vi "MultiTaskLassoCV.vi"(8 "error in":errorcluster) -> (0 "error out":errorcluster, 3 "out":refnum<class "MultiTaskLassoCV.lvclass">)   [LabVIEW 2020]
doc: "Multi-task Lasso model trained with L1/L2 mixed-norm as regularizer.\n\n See glossary entry for :term:`cross-validation estimator`.\n\n The optimization objective for MultiTaskLasso is::\n\n (1 / (2 * n_samples)) * ||Y - XW||^Fro_2 + alpha * ||W||_21\n\n Where::\n\n ||W||_21 = \\sum_i \\sqrt{\\sum_j w_{ij}^2}\n\n i.e. the sum of norm of each row.\n\n Read more in the :ref:`User Guide <multi_task_lasso>`.\n\n .. versionadded:: 0.15\n\n Parameters\n ----------\n eps : float, default=1e-3\n Length of the path. ``eps=1e-3`` means that\n ``alpha_min / alpha_max = 1e-3``.\n\n n_alphas : int, default=100\n Number of alphas along the regularization path.\n\n alphas : array-like, default=None\n List of alphas where to compute the models.\n If not provided, set automatically.\n\n fit_intercept : bool, default=True\n Whether to calculate the intercept for this model. If set\n to false, no intercept will be used in calculations\n (i.e. data is expected to be centered).\n\n normalize : bool, default=False\n This parameter is ignored when ``fit_intercept`` is set to False.\n If True, the regressors X will be normalized before regression by\n subtracting the mean and dividing by the l2-norm.\n If you wish to standardize, please use\n :class:`~sklearn.preprocessing.StandardScaler` before calling ``fit``\n on an estimator with ``normalize=False``.\n\n max_iter : int, default=1000\n The maximum number of iterations.\n\n tol : float, default=1e-4\n The tolerance for the optimization: if the updates are\n smaller than ``tol``, the optimization code checks the\n dual gap for optimality and continues until it is smaller\n than ``tol``.\n\n copy_X : bool, default=True\n If ``True``, X will be copied; else, it may be overwritten.\n\n cv : int, cross-validation generator or iterable, default=None\n Determines the cross-validation splitting strategy.\n Possible inputs for cv are:\n\n - None, to use the default 5-fold cross-validation,\n - int, to specify the number of folds.\n - :term:`CV splitter`,\n - An iterable yielding (train, test) splits as arrays of indices.\n\n For int/None inputs, :class:`KFold` is used.\n\n Refer :ref:`User Guide <cross_validation>` for the various\n cross-validation strategies that can be used here.\n\n .. versionchanged:: 0.22\n ``cv`` default value if None changed from 3-fold to 5-fold.\n\n verbose : bool or int, default=False\n Amount of verbosity.\n\n n_jobs : int, default=None\n Number of CPUs to use during the cross validation. Note that this is\n used only if multiple values for l1_ratio are given.\n ``None`` means 1 unless in a :obj:`joblib.parallel_backend` context.\n ``-1`` means using all processors. See :term:`Glossary <n_jobs>`\n for more details.\n\n random_state : int, RandomState instance, default=None\n The seed of the pseudo random number generator that selects a random\n feature to update. Used when ``selection`` == 'random'.\n Pass an int for reproducible output across multiple function calls.\n See :term:`Glossary <random_state>`.\n\n selection : {'cyclic', 'random'}, default='cyclic'\n If set to 'random', a random coefficient is updated every iteration\n rather than looping over features sequentially by default. This\n (setting to 'random') often leads to significantly faster convergence\n especially when tol is higher than 1e-4.\n\n Attributes\n ----------\n intercept_ : ndarray of shape (n_tasks,)\n Independent term in decision function.\n\n coef_ : ndarray of shape (n_tasks, n_features)\n Parameter vector (W in the cost function formula).\n Note that ``coef_`` stores the transpose of ``W``, ``W.T``.\n\n alpha_ : float\n The amount of penalization chosen by cross validation.\n\n mse_path_ : ndarray of shape (n_alphas, n_folds)\n Mean square error for the test set on each fold, varying alpha.\n\n alphas_ : ndarray of shape (n_alphas,)\n The grid of alphas used for fitting.\n\n n_iter_ : int\n Number of iterations run by the coordinate descent solver to reach\n the specified tolerance for the optimal alpha.\n\n dual_gap_ : float\n The dual gap at the end of the optimization for the optimal alpha.\n\n \nAvailable methods:\nGet Attributes\nGet Params\nSet Params"
uses:
  MultiTaskLassoCV.lvclass
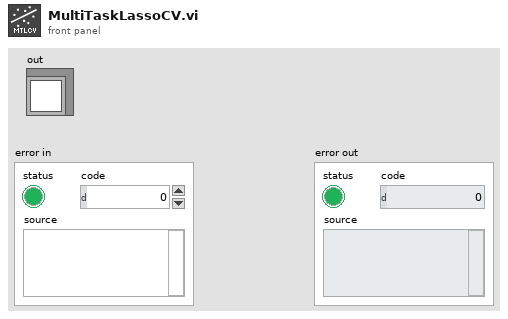
[diagram p1: front panel]
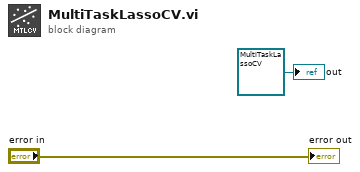
[diagram p0: block diagram]
diagram:
  "out" <- refnum<class "MultiTaskLassoCV.lvclass"> refnum ("model")
  "error out" <- "error in"
